vi "Report Data Update the Self.vi"(8 "error in (no error)":errorcluster, 10 "Report Data":T1={"Schema"="", "Test Socket"="", "Start Test Cycle"="", "Stop Test Cycle"="", "Test Mode"="", "Frame Type"="fe_frame_log"}, 11 "Test Info in":refnum<class "Test Info.lvclass">) -> (0 "error out":errorcluster, 3 "Test Info out":refnum<class "Test Info.lvclass">)   [LabVIEW 2023, in "Data Analysis.lvlib" / "Test Info.lvlib" / "Test Info.lvclass"]
uses:
  Test Info.lvclass
  Control/Report.ctl
  Test Info.lvclass/Test Info.ctl
  Data Analysis.lvlib
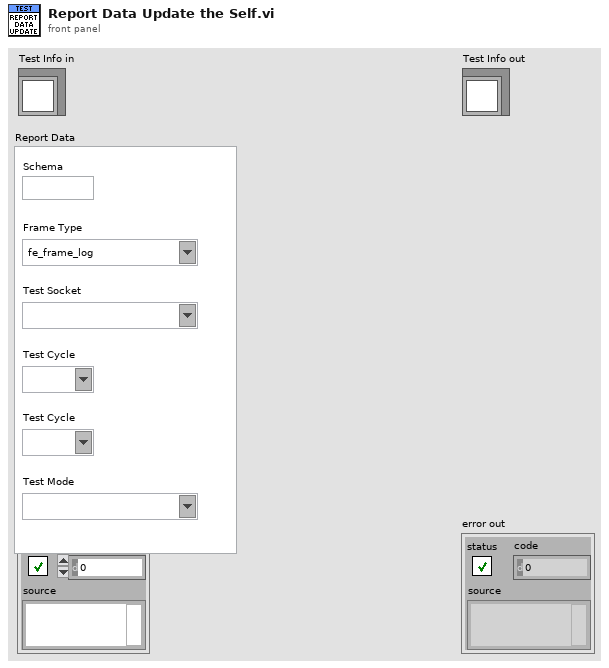
[diagram p1: front panel]
types:
  T1 = typedef "Data Analysis.lvlib/Report.ctl" = cluster{"Schema":string, "Test Socket":string, "Start Test Cycle":string, "Stop Test Cycle":string, "Test Mode":string, "Frame Type":string}
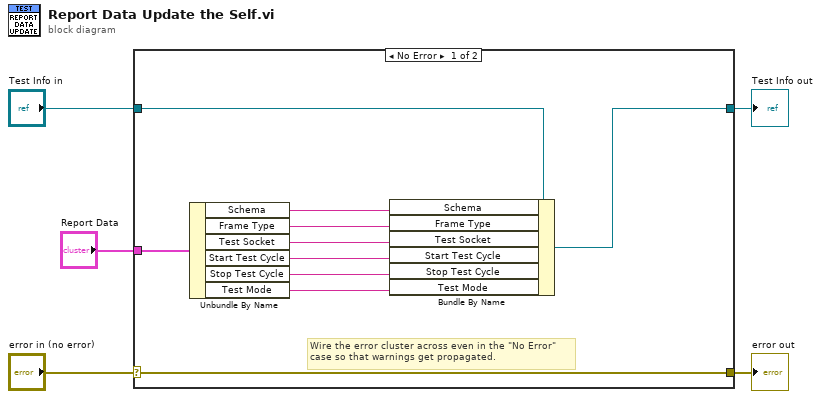
[diagram p0: block diagram]
diagram:
  n1 = case shown="No Error" "error in (no error)" {
    selector: "error in (no error)" -> [w15 w17]
    tunnel: [w15 w17] -> w4
    tunnel: [w14 w16] -> w2
    tunnel: "Test Info in" -> [w13 w16]
    tunnel: "Report Data" -> [w12 _]
    frame No Error {
      # "Wire the error cluster across even in the \"No Error\"\ncase so that warnings get propagated."
      n2 = Unbundle By Name(w12) -> ("Schema"=w6:string, "Frame Type"=w11:string, "Test Socket"=w10:string, "Start Test Cycle"=w9:string, "Stop Test Cycle"=w8:string, "Test Mode"=w7:string)
      n3 = Bundle By Name(cluster=w13, "Schema"=w6, "Frame Type"=w11, "Test Socket"=w10, "Start Test Cycle"=w9, "Stop Test Cycle"=w8, "Test Mode"=w7) -> (w14:refnum<class "Test Info.lvclass">)
    }
    frame Error {
    }
  }
  "error out" <- w4
  "Test Info out" <- w2
